vi "Record Call.vi"(8 "error in (no error)":errorcluster, 10 "This VI":refnum<vi>, 11 "Mock In":refnum<class "Mock.lvclass">) -> (0 "error out":errorcluster, 3 "Mock Out":refnum<class "Mock.lvclass">)   [LabVIEW 2020, in "Mock.lvclass"]
uses:
  Mock.lvclass
  Mock.lvclass/Mock.ctl
  Expectation/Expectation.lvclass
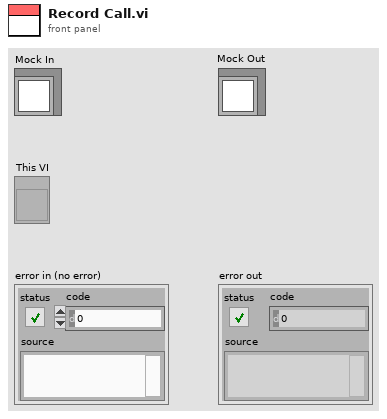
[diagram p1: front panel]
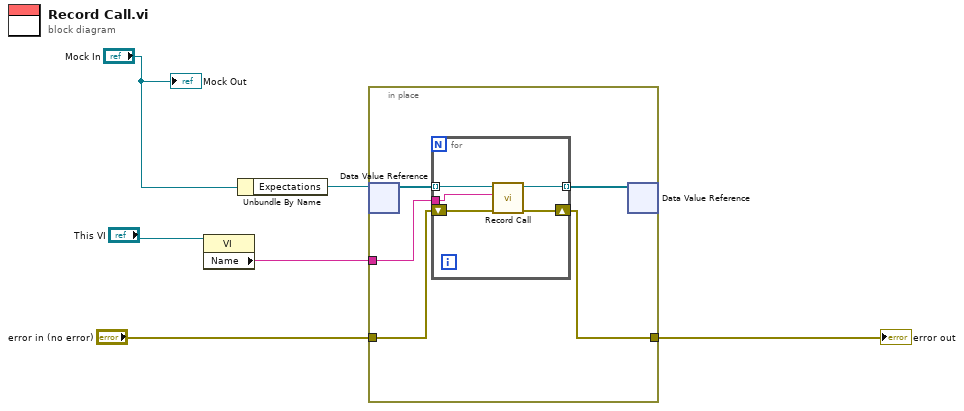
[diagram p0: block diagram]
diagram:
  n1 = property class="VI"(reference="This VI") -> ("Name"=w5:string)  [unwired: 1 in, 2 out]
  n2 = Unbundle By Name("Mock In") -> ("Expectations"=w6:refnum<data-value>)
  n3 = in-place {
    in-place-border: [w11] -> w3
    in-place-border: "error in (no error)" -> [w10]
    in-place-border: w5 -> [w9]
    n4 = in-place-dvr #1(w6) -> (w8:refnum<class "Expectation.lvclass">[])  [unwired: 1 out]
    n5 = for {
      tunnel: w8 -> [w16] mode=indexing
      tunnel: [w15] -> w7 mode=indexing
      shift-right: [w14] -> w11
      shift-left: w10 -> [w13]
      tunnel: w9 -> [w12]
      n6 = call-dynamic "Record Call.vi"("error in (no error)"=w13, "VI Name"=w12, "Expectation in"=w16) -> ("error out"=w14:errorcluster, "Expectation out"=w15:refnum<class "Expectation.lvclass">)  [unwired: 7 in]
    }
    n7 = in-place-dvr #1(w7) -> ()  [unwired: 2 out]
  }
  "error out" <- w3
  "Mock Out" <- "Mock In"
